vi "Sam's Basic Driver for Encapsulation Station.vi"(8 "error in (no error)":errorcluster, 9 "Parameter Array":dbl[](array[numeric]), 10 "Combo Box":string(combo), 11 "VISA resource name":refnum<visa-resource-name>) -> (0 "error out":errorcluster, 2 "return count 2":u32, 3 "read buffer 2":string)   [LabVIEW 2011]
uses:
  <vilib>/Instr/_visa.llb/VISA Configure Serial Port (Instr).vi
panel:
  out "byte count 2":u32
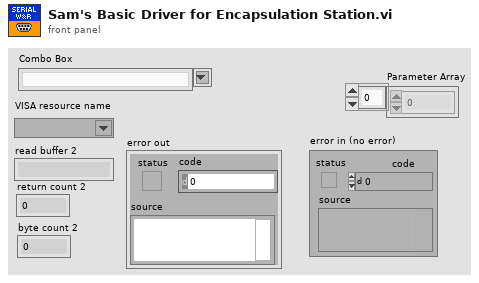
[diagram p1: front panel]
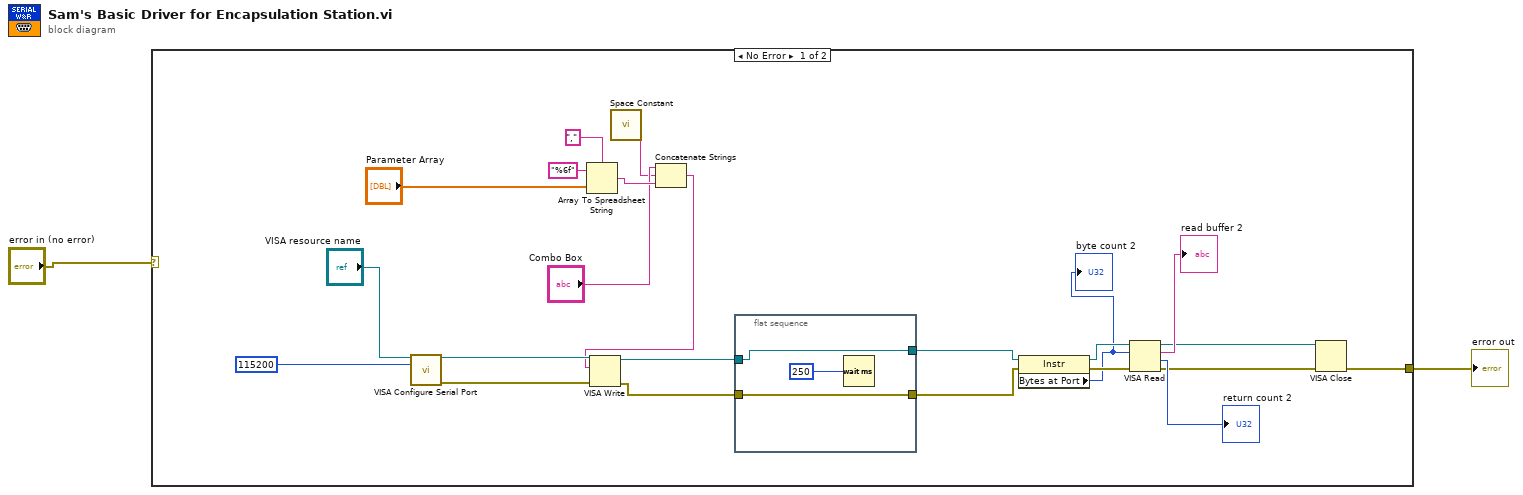
[diagram p0: block diagram]
diagram:
  n1 = case shown="No Error" "error in (no error)" {
    selector: "error in (no error)" -> [_ w29]
    tunnel: [w23 w29] -> w2
    frame No Error {
      n2 = call-poly "VISA Configure Serial Port"("VISA resource name"="VISA resource name", "baud rate (9600)"=u32 115200) -> ("VISA resource name out"=w22:refnum<visa-resource-name>, "error out"=w21:errorcluster)  [unwired: 12 in]
      n3 = Array To Spreadsheet String(delimiter (Tab)=",", array="Parameter Array", 3:"%6f" ("format string")) -> (spreadsheet string=w6:string)
      n4 = call <vilib>:"Space Constant.vi"() -> ("String"=w4:string)
      n5 = Concatenate Strings("Combo Box", w4, w6) -> (w3:string)
      n6 = VISA Write(VISA resource name=w22, write buffer=w3, error in (no error)=w21) -> (VISA resource name out=w20:refnum<visa-resource-name>, error out=w19:errorcluster)  [unwired: 1 out]
      n7 = flat-sequence {
        tunnel: w20 -> [w27]
        tunnel: w19 -> [w26]
        tunnel: [w27] -> w11
        tunnel: [w26] -> w10
        frame #0 {
          n8 = Wait (ms)(milliseconds to wait=u32 250) -> ()  [unwired: 1 out]
        }
      }
      n9 = property class="Instr"(reference=w11, error in=w10) -> (reference out=w17:refnum<visa-resource-name>, error out=w18:errorcluster, "Bytes at Port"=w14:u32)
      "byte count 2" <- w14
      n10 = VISA Read(VISA resource name=w17, byte count=w14, error in (no error)=w18) -> (VISA resource name out=w13:refnum<visa-resource-name>, read buffer=→"read buffer 2":string, return count=→"return count 2":u32, error out=w12:errorcluster)
      n11 = VISA Close(VISA resource name=w13, error in (no error)=w12) -> (error out=w23:errorcluster)
    }
    frame Error {
    }
  }
  "error out" <- w2
